vi "Set Player Ship.vi"(8 "error in (no error)":errorcluster, 10 "Player Ship":T1, 11 "Main Controller Actor in":refnum<class "Main Controller Actor.lvclass">) -> (0 "error out":errorcluster, 3 "Main Controller Actor out":refnum<class "Main Controller Actor.lvclass">)   [LabVIEW 2021, in "Main Controller Actor.lvclass"]
uses:
  Main Controller Actor.lvclass
  Main Controller Actor.lvclass/Main Controller Actor.ctl
  Ships/Arilou/Arilou.lvclass
  Ships/Chmmr/Chmmr.lvclass
  Ships/Kohrah/Kohrah.lvclass
  Ships/Slylandro/Slylandro.lvclass
  Ship/Ship.lvclass
  Renderer/Renderer.lvclass
  Element/Element.lvclass
  Element/Player Type.ctl
  Globals.vi
  Player.ctl
  Ship.ctl
  Player Ship.ctl
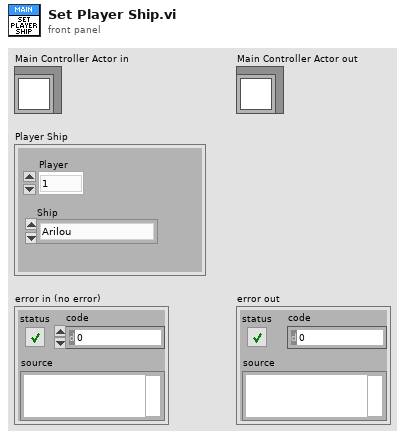
[diagram p1: front panel]
types:
  T1 = typedef "Main Controller Actor.lvclass/Player Ship.ctl" = cluster{"Player":T2, "Ship":T3}
  T2 = typedef "Main Controller Actor.lvclass/Player.ctl" = enum16{"1", "2"}
  T3 = typedef "Main Controller Actor.lvclass/Ship.ctl" = enum16{"Arilou", "Chmmr", "Kohrah", "Slylandro"}
  T4 = typedef "Element.lvclass/Player Type.ctl" = enum16{"Neutral", "Player 1", "Player 2"}
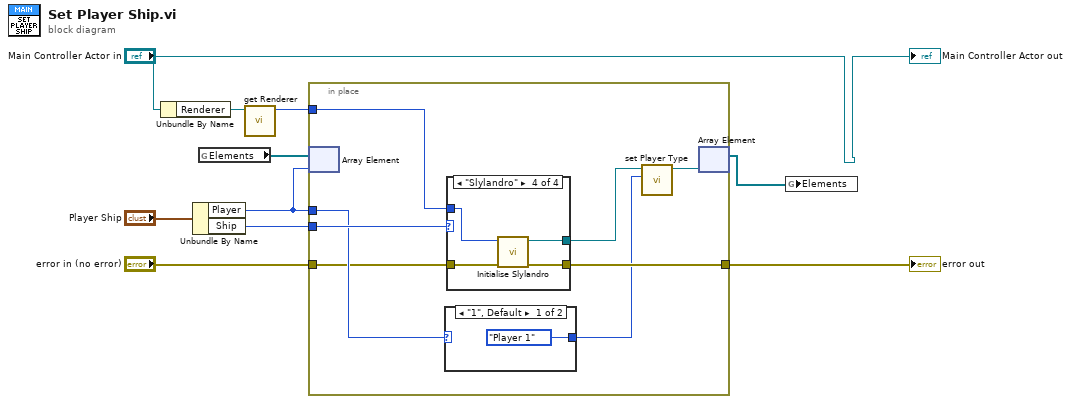
[diagram p0: block diagram]
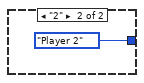
[diagram p2: hidden frame]
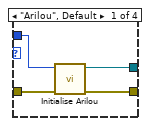
[diagram p3: hidden frame]
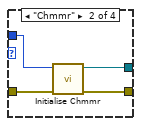
[diagram p4: hidden frame]
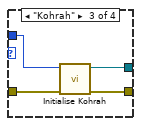
[diagram p5: hidden frame]
diagram:
  n1 = Unbundle By Name("Main Controller Actor in") -> ("Renderer"=w1:refnum<class "Renderer.lvclass">)
  n2 = Unbundle By Name("Player Ship") -> ("Player"=w10:T2, "Ship"=w9:T3)
  n3 = global read "Globals.vi" "Elements"() -> (w5:refnum<class "Element.lvclass">[])
  n4 = call-dynamic "get Renderer.vi"("Renderer in"=w1) -> ("Renderer"=w2:u32)  [unwired: 10 in]
  n5 = in-place {
    in-place-border: w10 -> [w14]
    in-place-border: "error in (no error)" -> [w12]
    in-place-border: [w15] -> w8
    in-place-border: w9 -> [w18]
    in-place-border: w2 -> [w13]
    n6 = in-place-array #1(w5, w10) -> ()  [unwired: 1 out]
    n7 = case shown="\"1\", Default" w14 {
      tunnel: [Player_Type."Player 1" ("Player Type") Player_Type."Player 2" ("Player Type")] -> w11
      frame "1", Default {
      }
      frame "2" {
      }
    }
    n8 = case shown="\"Slylandro\"" w18 {
      tunnel: w12 -> [w24 w28 w32 w36]
      tunnel: [w23 w27 w31 w35] -> w15
      tunnel: [w22 w26 w30 w34] -> w16
      tunnel: w13 -> [w21 w25 w29 w33]
      frame "Arilou", Default {
        n9 = call "Initialise Arilou.vi"("error in (no error)"=w24, "Renderer"=w21) -> ("error out"=w23:errorcluster, "Ship out"=w22:refnum<class "Arilou.lvclass">)  [unwired: 8 in]
      }
      frame "Chmmr" {
        n10 = call "Initialise Chmmr.vi"("error in (no error)"=w28, "Renderer"=w25) -> ("error out"=w27:errorcluster, "Ship out"=w26:refnum<class "Chmmr.lvclass">)  [unwired: 7 in, 1 out]
      }
      frame "Kohrah" {
        n11 = call "Initialise Kohrah.vi"("error in (no error)"=w32, "Renderer"=w29) -> ("error out"=w31:errorcluster, "Ship out"=w30:refnum<class "Kohrah.lvclass">)  [unwired: 8 in]
      }
      frame "Slylandro" {
        n12 = call "Initialise Slylandro.vi"("error in (no error)"=w36, "Renderer"=w33) -> ("error out"=w35:errorcluster, "Ship out"=w34:refnum<class "Slylandro.lvclass">)  [unwired: 8 in]
      }
    }
    n13 = call "set Player Type.vi"("Player Type"=w11, "Element in"=w16) -> ("Element out"=w17:refnum<class "Ship.lvclass">)  [unwired: 9 in]
    n14 = in-place-array #1(w17) -> (w4:refnum<class "Element.lvclass">[])  [unwired: 1 out]
  }
  "error out" <- w8
  n15 = global write "Globals.vi" "Elements"(w4) -> ()
  "Main Controller Actor out" <- "Main Controller Actor in"
